vi "CommutationSignal.vi"(10 "Array in":dbl[][](array[numeric]), 11 "Treshold":dbl) -> (3 "Array out":i32[](array[numeric]))   [LabVIEW 2020]
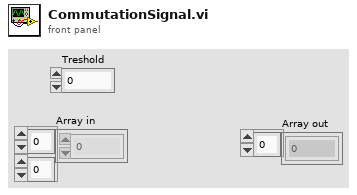
[diagram p1: front panel]
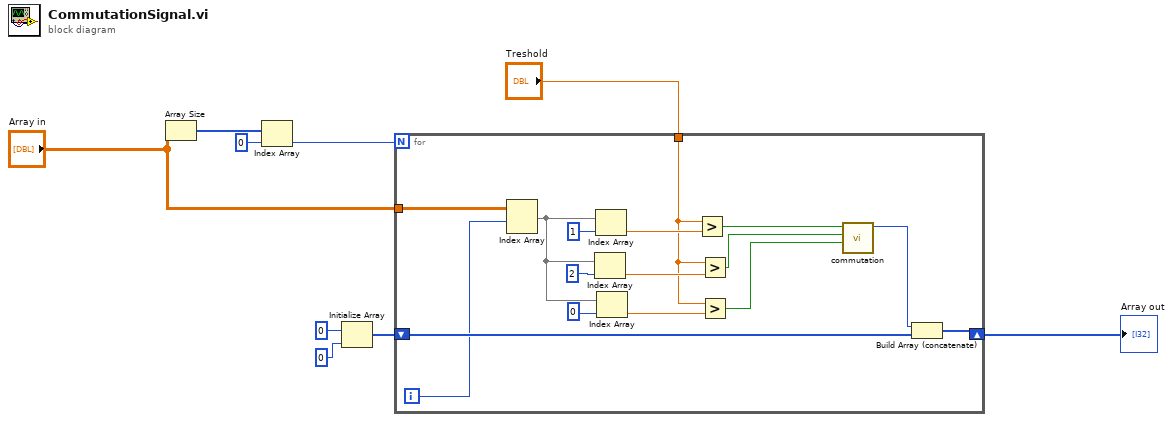
[diagram p0: block diagram]
diagram:
  n1 = Array Size(array="Array in") -> (size(s)=w5:i32[])
  n2 = Index Array(array=w5, index=0) -> (element=w2:i32)
  n3 = Initialize Array(0, 0 ("dimension size")) -> (w7:i32[])
  n4 = for {
    N: w2 -> [_]
    tunnel: "Array in" -> [w25]
    shift-right: [w13] -> w9
    shift-left: w7 -> [w14]
    tunnel: "Treshold" -> [w10]
    i -> [w11]
    n5 = Index Array(array=w25, index (row)=w11) -> (element=w20:dbl[])  [unwired: 1 in]
    n6 = Index Array(array=w20, index=2) -> (element=w19:dbl)
    n7 = Index Array(array=w20, index=1) -> (element=w23:dbl)
    n8 = Index Array(array=w20, index=0) -> (element=w18:dbl)
    n9 = Greater?(x=w10, y=w23) -> (0:w17:bool)
    n10 = Greater?(x=w10, y=w19) -> (0:w16:bool)
    n11 = Greater?(x=w10, y=w18) -> (0:w15:bool)
    n12 = call "commutation.vi"("Hall C"=w15, "Hall B"=w16, "Hall A"=w17) -> ("Commutation"=w12:i32)  [unwired: 8 in]
    n13 = Build Array (concatenate)(w12, w14) -> (w13:i32[])
  }
  "Array out" <- w9
